vi "S3859061_Task3.vi"() -> ()   [LabVIEW 2020]
panel:
  out "quotient":dbl
  out "remainder":dbl
  out "odd sum":dbl
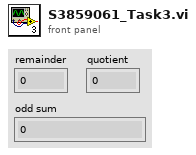
[diagram p1: front panel]
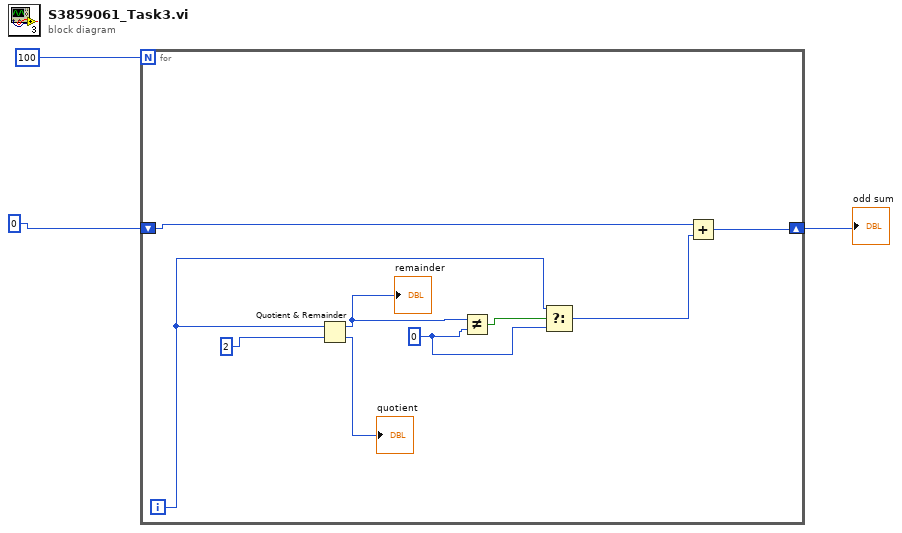
[diagram p0: block diagram]
diagram:
  n1 = for {
    N: 100 -> [_]
    shift-right: [w4] -> w1
    shift-left: 0 -> [w6]
    i -> [w8]
    w7 = 0
    n2 = Quotient & Remainder(x=w8, y=2) -> (x-y*floor(x/y)=w10:i32, floor(x/y)=→"quotient":i32)
    "remainder" <- w10
    n3 = Not Equal?(x=w10, y=w7) -> (x != y?=w9:bool)
    n4 = Select(t=w8, s=w9, f=w7) -> (s? t:f=w5:i32)
    n5 = Add(x=w6, y=w5) -> (x+y=w4:i32)
  }
  "odd sum" <- w1
